vi "Date Type Format String Mapping.vi"(10 "Type Formatting":T1) -> (2 "Type Formatting populated":T1)   [LabVIEW 2011]
uses:
  Options API/Private/EasyXML Options - Type Formatting Cluster.ctl
  Type Defs/Formatting Data Type -- Enum.ctl
panel:
  # "OpenG Date Type Format String Mapping.vi  - Gets the format strings for all valid data types\n\nCopyright (C) 2003 Jim Kring jim@jimkring.com\n\nThis library is free software; you can redistribute it and/or\nmodify it under the terms of the GNU Lesser General Public\nLicense as published by the Free Software Foundation; either\nversion 2.1 of the License, or (at your option) any later version.\nThis library is distributed in the hope that it will be useful,\nbut WITHOUT ANY WARRANTY; without even the implied warranty of\nMERCHANTABILITY or FITNESS FOR A PARTICULAR PURPOSE. See the GNU\nLesser General Public License for more details.\nYou should have received a copy of the GNU Lesser General Public\nLicense along with this library; if not, write to the Free Software\nFoundation, Inc., 59 Temple Place, Suite 330, Boston, MA 02111-1307 USA"
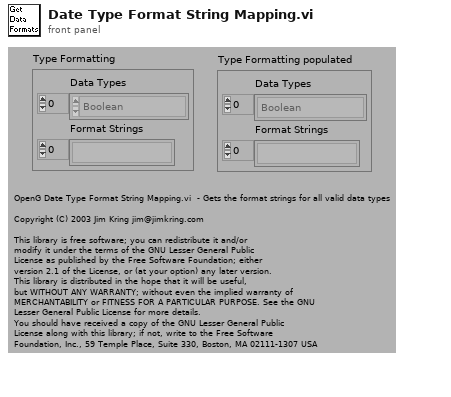
[diagram p1: front panel]
types:
  T1 = typedef "EasyXML Options - Type Formatting Cluster.ctl" = cluster{"Data Types":T2[], "Format Strings":string[]}
  T2 = typedef "Formatting Data Type -- Enum.ctl" = enum16{"<unknown>", "Cluster", "Array", "String", "Path", "Boolean", "Time Stamp", "Enum", "Numeric - EXT", "Numeric - DBL", "Numeric - SGL", "Numeric - I64", "Numeric - I32", "Numeric - I16", "Numeric - I8", "Numeric - U64", "Numeric - U32", "Numeric - U16", "Numeric - U8", "Numeric - CXT", "Numeric - CDB", "Numeric - CSG", "VISA Resource"}
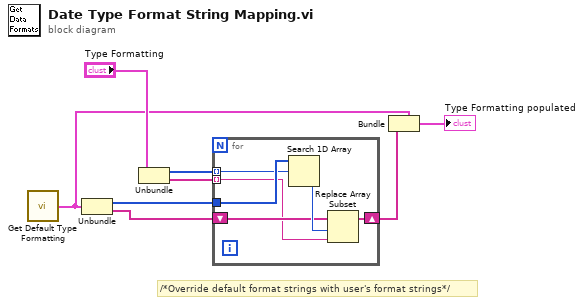
[diagram p0: block diagram]
diagram:
  # "/*Override default format strings with user's format strings*/"
  n1 = call "Get Default Type Formatting.vi"() -> ("Default Type Formatting"=w3:T1)
  n2 = Unbundle(w3) -> ("Data Types"=w2:T2[], "Format Strings"=w1:string[])
  n3 = Unbundle("Type Formatting") -> ("Data Types"=w6:T2[], "Format Strings"=w7:string[])
  n4 = for {
    shift-right: [w12] -> w8
    shift-left: w1 -> [w13]
    tunnel: w2 -> [w11]
    tunnel: w7 -> [w10] mode=indexing
    tunnel: w6 -> [w9] mode=indexing
    n5 = Search 1D Array(1D array=w11, element=w9) -> (index of element=w14:i32)  [unwired: 1 in]
    n6 = Replace Array Subset(array=w13, new element=w10, index=w14) -> (w12:string[])
  }
  n7 = Bundle(cluster=w3, "Format Strings"=w8) -> (→"Type Formatting populated":T1)  [unwired: 1 in]
